vi "Test.vi"   [LabVIEW 2013]
doc: "This VI is called when test mode begins, and will automatically be terminated when it ends. You can add manual or automatic tests and invoke them from the dashboard."
uses:
  Robot Global Data.vi
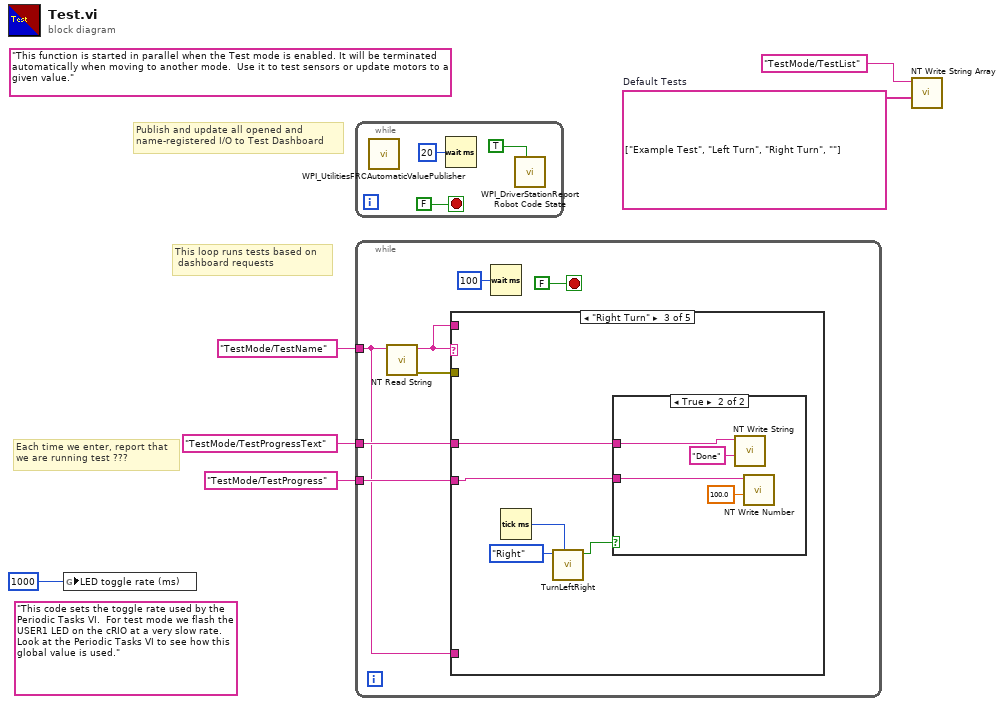
[diagram p0: block diagram]
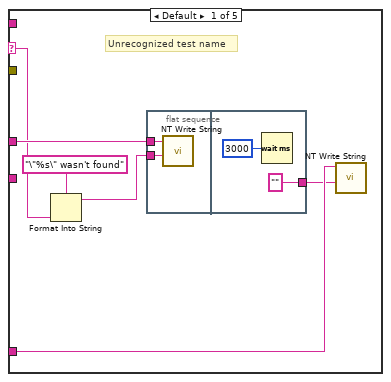
[diagram p2: hidden frame]
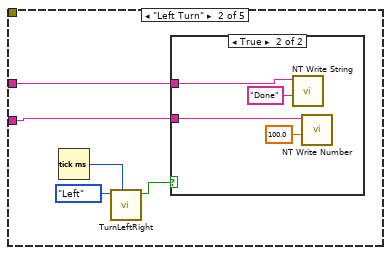
[diagram p3: hidden frame]
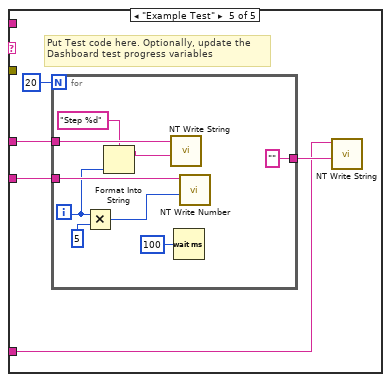
[diagram p7: hidden frame]
diagram:
  w2 = string[] ["Example Test", "Left Turn", "Right Turn", ""]  # Default Tests
  (unwired) "This code sets the toggle rate used by the Periodic Tasks VI.  For test mode we flash the USER1 LED on the cRIO at a very slow rate.  Look at the Periodic Tasks VI to see how this global value is used."
  (unwired) "This function is started in parallel when the Test mode is enabled. It will be terminated automatically when moving to another mode.  Use it to test sensors or update motors to a given value."
  # "This loop runs tests based on \n dashboard requests"
  # "Publish and update all opened and\nname-registered I/O to Test Dashboard"
  # "Each time we enter, report that\nwe are running test ???"
  n1 = global write "Robot Global Data.vi" "LED toggle rate (ms)"(u32 1000 ("LED ms toggle rate")) -> ()
  n2 = while {
    stop <- FALSE stop-if-true
    n3 = call <vilib>:"WPI_UtilitiesFRCAutomaticValuePublisher.vi"() -> ()  [unwired: 12 in]
    n4 = Wait (ms)(milliseconds to wait=u32 20) -> ()  [unwired: 1 out]
    n5 = call <vilib>:"WPI_DriverStationReport Robot Code State.vi"("Test"=TRUE ("Autonomous")) -> ()  [unwired: 10 in, 1 out]
  }
  n6 = while {
    tunnel: "TestMode/TestName" ("Name") -> [w11]
    tunnel: "TestMode/TestProgressText" ("Name") -> [w14]
    tunnel: "TestMode/TestProgress" ("Name") -> [w13]
    stop <- FALSE stop-if-true
    n7 = call <vilib>:"NT Read String.vi"("Name"=w11) -> ("error out"=w10:errorcluster, "String"=w12:string)  [unwired: 9 in]
    n8 = case shown="\"Right Turn\"" w12 {
      selector: w12 -> [w21 _ _ _ _]
      tunnel: w11 -> [w18 _ _ _ w45]
      tunnel: w14 -> [w22 w30 w39 _ w48]
      tunnel: w13 -> [_ w29 w38 _ w49]
      tunnel: w12 -> [_ _ _ _ _]
      tunnel: w10 -> [_ _ _ _ _]
      frame Default {
        # "Unrecognized test name"
        n9 = Format Into String(format string="\"%s\" wasn't found" ("Name"), w21) -> (resulting string=w20:string)  [unwired: 2 in, 1 out]
        n10 = flat-sequence {
          tunnel: w22 -> [w23]
          tunnel: w20 -> [w24]
          tunnel: ["" ("Name")] -> w17
          frame #0 {
            n11 = call <vilib>:"NT Write String.vi"("String"=w24, "Name"=w23) -> ()  [unwired: 9 in, 1 out]
          }
          frame #1 {
            n12 = Wait (ms)(milliseconds to wait=u32 3000) -> ()  [unwired: 1 out]
          }
        }
        n13 = call <vilib>:"NT Write String.vi"("String"=w17, "Name"=w18) -> ()  [unwired: 9 in, 1 out]
      }
      frame "Left Turn" {
        n14 = Tick Count (ms)() -> (millisecond timer value=w31:u32)
        n15 = call "TurnLeftRight.vi"("Start time"=w31, "Left/Right"=enum16{"Left", "Right", ""}."Left") -> ("Done"=w27:bool)  [unwired: 9 in]
        n16 = case shown="True" w27 {
          tunnel: w30 -> [_ w35]
          tunnel: w29 -> [_ w34]
          frame False {
          }
          frame True {
            n17 = call <vilib>:"NT Write String.vi"("String"="Done", "Name"=w35) -> ()  [unwired: 9 in, 1 out]
            n18 = call <vilib>:"NT Write Number.vi"("Numeric"=100.0, "Name"=w34) -> ()  [unwired: 9 in, 1 out]
          }
        }
      }
      frame "Right Turn" {
        n19 = Tick Count (ms)() -> (millisecond timer value=w40:u32)
        n20 = call "TurnLeftRight.vi"("Start time"=w40, "Left/Right"=enum16{"Left", "Right", ""}."Right") -> ("Done"=w36:bool)  [unwired: 9 in]
        n21 = case shown="True" w36 {
          tunnel: w39 -> [_ w44]
          tunnel: w38 -> [_ w43]
          frame False {
          }
          frame True {
            n22 = call <vilib>:"NT Write String.vi"("String"="Done", "Name"=w44) -> ()  [unwired: 9 in, 1 out]
            n23 = call <vilib>:"NT Write Number.vi"("Numeric"=100.0, "Name"=w43) -> ()  [unwired: 9 in, 1 out]
          }
        }
      }
      frame ? {
      }
      frame "Example Test" {
        # "Put Test code here. Optionally, update the\nDashboard test progress variables"
        n24 = for {
          N: 20 -> [_]
          tunnel: w49 -> [w58]
          tunnel: w48 -> [w56]
          tunnel: ["" ("String")] -> w46
          i -> [w53]
          n25 = Multiply(x=w53, y=u32 5 ("milliseconds to wait")) -> (x*y=w54:u32)
          n26 = Format Into String(format string="Step %d", w53) -> (resulting string=w51:string)  [unwired: 2 in, 1 out]
          n27 = call <vilib>:"NT Write String.vi"("String"=w51, "Name"=w56) -> ()  [unwired: 9 in, 1 out]
          n28 = Wait (ms)(milliseconds to wait=u32 100) -> ()  [unwired: 1 out]
          n29 = call <vilib>:"NT Write Number.vi"("Numeric"=w54, "Name"=w58) -> ()  [unwired: 9 in, 1 out]
        }
        n30 = call <vilib>:"NT Write String.vi"("String"=w46, "Name"=w45) -> ()  [unwired: 9 in, 1 out]
      }
    }
    n31 = Wait (ms)(milliseconds to wait=u32 100) -> ()  [unwired: 1 out]
  }
  n32 = call <vilib>:"NT Write String Array.vi"("String Array"=w2, "Name"="TestMode/TestList") -> ()  [unwired: 9 in, 1 out]
